vi "Shooter.vi"   [LabVIEW 2020]
uses:
  <vilib>/Rock Robotics/WPI/Utilities/WPI_GetSetVariantRefNum.vi
types:
  T1 = typedef "WPI_JoystickDevRef.ctl" = cluster{"Device":T2}
  T2 = typedef "WPI_JoystickDeviceEnum.ctl" = enum16{"USB 0", "USB 1", "USB 2", "USB 3", "USB 4", "USB 5"}
  T3 = typedef "WPI_MotorControlDeviceRef.ctl" = cluster{"DeviceStatus":errorcluster, "Type":T4, "PWM":cluster{"PWM Channel":T5, "DeadBand":T6}, "CAN":cluster{"Device Number":u8, "SetOutput VI Ref":variant, "GetOutput VI Ref":variant, "Enable VI Ref":variant, "Disable VI Ref":variant, "Data":variant}, "Invert":bool, "DIO PWM":cluster{"PWM \"Enable\" Channel":T5, "DIOChannel":T7, "PWM Rate":dbl}}
  T4 = typedef "WPI_MotorControlType.ctl" = enum16{"PWM", "CAN", "DIO PWM"}
  T5 = typedef "FPGA_DIOPWMChannel.ctl" = enum8{"PWM 0", "PWM 1", "PWM 2", "PWM 3", "PWM 4", "PWM 5", "PWM 6", "PWM 7", "PWM 8", "PWM 9", "PWM MXP 0", "PWM MXP 1", "PWM MXP 2", "PWM MXP 3", "PWM MXP 4", "PWM MXP 5", "PWM MXP 6", "PWM MXP 7", "PWM MXP 8", "PWM MXP 9", "Invalid"}
  T6 = typedef "WPI_PWMDeadband.ctl" = cluster{"Name":string, "maxPositivePwm":i32, "minPositivePwm":i32, "centerPwm":i32, "maxNegativePwm":i32, "minNegativePwm":i32, "angularRange":u16}
  T7 = typedef "FPGA_DIOChannel.ctl" = enum8{"DIO 0", "DIO 1", "DIO 2", "DIO 3", "DIO 4", "DIO 5", "DIO 6", "DIO 7", "DIO 8", "DIO 9", "DIO MXP 0", "DIO MXP 1", "DIO MXP 2", "DIO MXP 3", "DIO MXP 4", "DIO MXP 5", "DIO MXP 6", "DIO MXP 7", "DIO MXP 8", "DIO MXP 9", "DIO MXP 10", "DIO MXP 11", "DIO MXP 12", "DIO MXP 13", "DIO MXP 14", "DIO MXP 15", "SPI Port CS1", "SPI Port CS2", "SPI Port CS3", "SPI Port MISO", "SPI Port MOSI", "Invalid"}
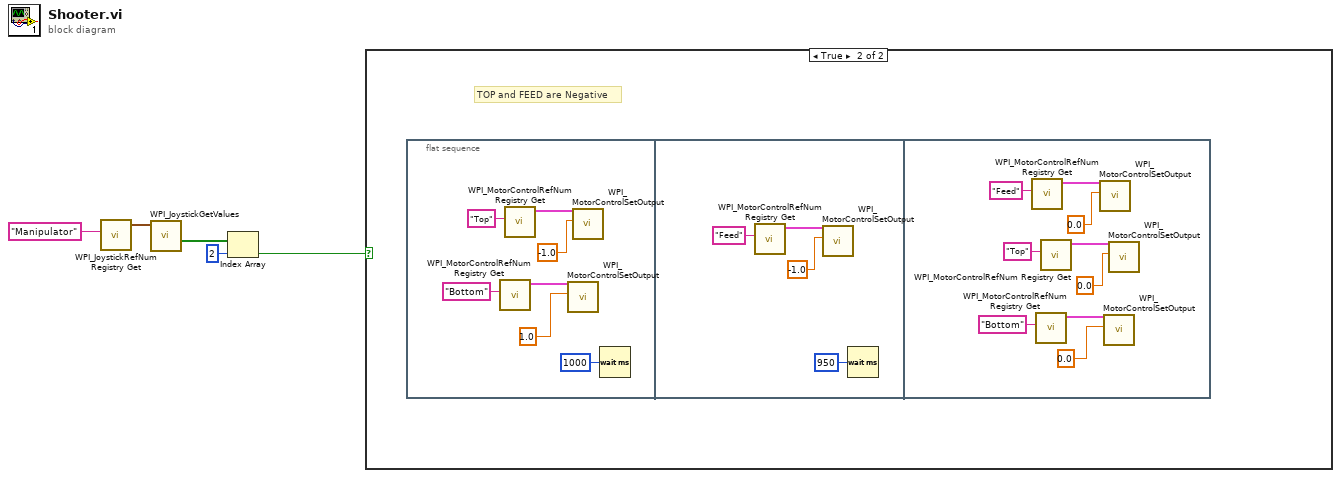
[diagram p0: block diagram]
diagram:
  n1 = call <vilib>:"WPI_JoystickRefNum Registry Get.vi"("refnum name"="Manipulator") -> ("JoystickDevRef"=w5:T1)  [unwired: 9 in, 1 out]
  n2 = call <vilib>:"WPI_JoystickGetValues.vi"("JoystickDevRef"=w5) -> ("Buttons"=w3:bool[])  [unwired: 6 in, 4 out]
  n3 = Index Array(array=w3, index=2) -> (element=w1:bool)
  n4 = case shown="True" w1 {
    frame False {
    }
    frame True {
      # "TOP and FEED are Negative"
      n5 = flat-sequence {
        frame #0 {
          n6 = call <vilib>:"WPI_MotorControlRefNum Registry Get.vi"("refnum name"="Bottom") -> ("MotorControlDevRef"=w9:T3)  [unwired: 9 in, 1 out]
          n7 = call <vilib>:"WPI_MotorControlRefNum Registry Get.vi"("refnum name"="Top") -> ("MotorControlDevRef"=w11:T3)  [unwired: 9 in, 1 out]
          n8 = call <vilib>:"WPI_MotorControlSetOutput.vi"("Output"=1.0, "MotorControlDevRef"=w9) -> ()  [unwired: 7 in, 3 out]
          n9 = call <vilib>:"WPI_MotorControlSetOutput.vi"("Output"=-1.0, "MotorControlDevRef"=w11) -> ()  [unwired: 7 in, 3 out]
          n10 = Wait (ms)(milliseconds to wait=u32 1000) -> ()  [unwired: 1 out]
        }
        frame #1 {
          n11 = call <vilib>:"WPI_MotorControlRefNum Registry Get.vi"("refnum name"="Feed") -> ("MotorControlDevRef"=w15:T3)  [unwired: 9 in, 1 out]
          n12 = call <vilib>:"WPI_MotorControlSetOutput.vi"("Output"=-1.0, "MotorControlDevRef"=w15) -> ()  [unwired: 7 in, 3 out]
          n13 = Wait (ms)(milliseconds to wait=u32 950) -> ()  [unwired: 1 out]
        }
        frame #2 {
          n14 = call <vilib>:"WPI_MotorControlRefNum Registry Get.vi"("refnum name"="Feed") -> ("MotorControlDevRef"=w24:T3)  [unwired: 9 in, 1 out]
          n15 = call <vilib>:"WPI_MotorControlRefNum Registry Get.vi"("refnum name"="Bottom") -> ("MotorControlDevRef"=w20:T3)  [unwired: 9 in, 1 out]
          n16 = call <vilib>:"WPI_MotorControlRefNum Registry Get.vi"("refnum name"="Top") -> ("MotorControlDevRef"=w18:T3)  [unwired: 9 in, 1 out]
          n17 = call <vilib>:"WPI_MotorControlSetOutput.vi"("Output"=0.0, "MotorControlDevRef"=w24) -> ()  [unwired: 7 in, 3 out]
          n18 = call <vilib>:"WPI_MotorControlSetOutput.vi"("Output"=0.0, "MotorControlDevRef"=w20) -> ()  [unwired: 7 in, 3 out]
          n19 = call <vilib>:"WPI_MotorControlSetOutput.vi"("Output"=0.0, "MotorControlDevRef"=w18) -> ()  [unwired: 7 in, 3 out]
        }
      }
    }
  }
